vi "move_to_absolute_position.vi"(0 "device_index (in) [0=def]":i32, 5 "Error In":errorcluster) -> (19 "Error Out":errorcluster)   [LabVIEW 2013, in "examples.lvlib"]
doc: "Produced By:\n\n<B>Kod Integrations, LLC</B>\n4835 Marianne Drive\nMount Airy, MD 21771\nhttp://www.kodintegrations.com\nemail: info@kodintegrations.com\nphone: (240) 687-1288"
uses:
  libraries/examples.lvlib
  classes/Controller/_Controller.lvclass
  common/controls/motor_enabled_state_axes_group.ctl
  libraries/common.lvlib
  common/controls/axis.ctl
  common/controls/movement_item.ctl
panel:
  out "response":string
  out "success?":bool
  in  "target_value (in)":i32
  in  "axis (def=X)":T1
  in  "clear_buffer? (T)":bool=TRUE
  # "instructions:\n\nAt the specified device index, enter a target position\nvalue and (for multi-controller applications only) a\nspecific axis and run the VI.\n\nNOTE: This example VI makes an attempt to enable\nthe motor at the targeted axis.  If left disabled, the\nmove command will appear to be successful, but\nthe motor physically does not respond."
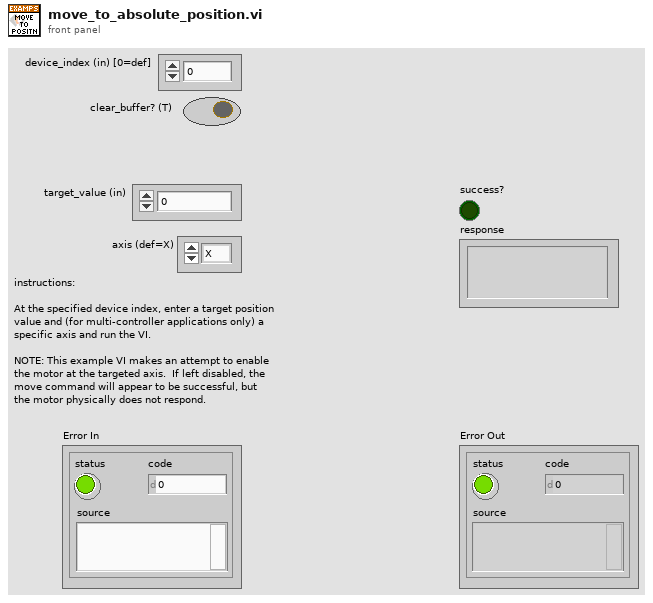
[diagram p1: front panel]
types:
  T1 = typedef "common.lvlib/axis.ctl" = enum16{"X", "Y", "Z", "U"}
  T2 = typedef "common.lvlib/movement_item.ctl" = cluster{"axis":T1, "target":i32}
  T3 = typedef "common.lvlib/motor_enabled_state_axes_group.ctl" = cluster{"x-axis":bool, "y-axis":bool, "z-axis":bool, "u-axis":bool}
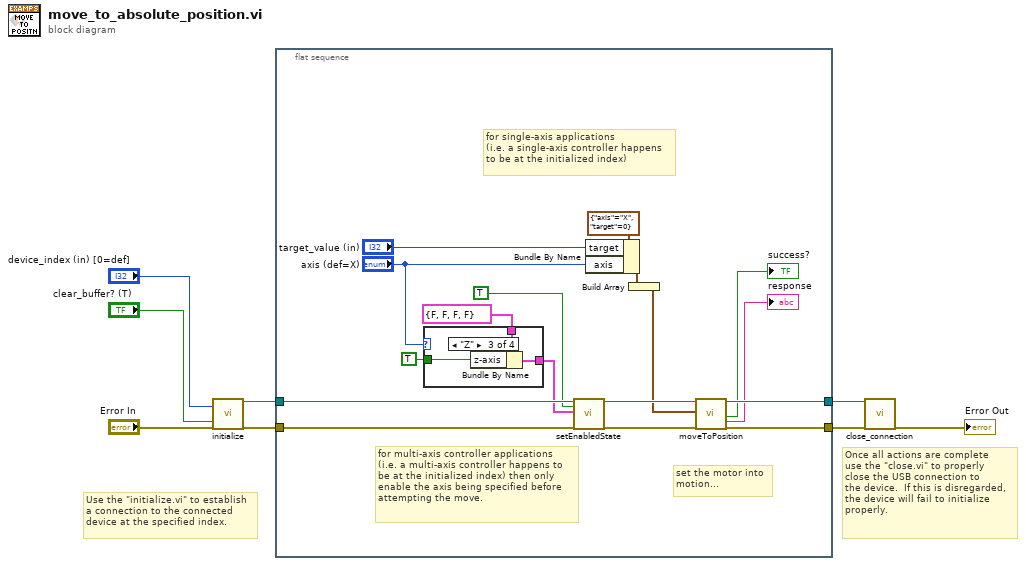
[diagram p0: block diagram]
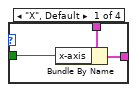
[diagram p2: hidden frame]
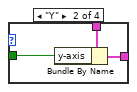
[diagram p3: hidden frame]
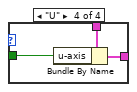
[diagram p4: hidden frame]
diagram:
  # "Once all actions are complete\nuse the \"close.vi\" to properly\nclose the USB connection to \nthe device.  If this is disregarded,\nthe device will fail to initialize \nproperly."
  # "Use the \"initialize.vi\" to establish\na connection to the connected\ndevice at the specified index."
  n1 = call "initialize.vi"("device_index (in) [0=def]"="device_index (in) [0=def]", "clear_buffer? (T)"="clear_buffer? (T)", "error in (no error)"="Error In") -> ("reference (out)"=w5:refnum<class "_Controller.lvclass">, "error out"=w4:errorcluster)  [unwired: 15 in]
  n2 = flat-sequence {
    tunnel: w5 -> [w21]
    tunnel: w4 -> [w20]
    tunnel: [w25] -> w3
    tunnel: [w24] -> w2
    frame #0 {
      # "set the motor into\nmotion..."
      # "for single-axis applications\n(i.e. a single-axis controller happens\nto be at the initialized index)"
      # "for multi-axis controller applications\n(i.e. a multi-axis controller happens to\nbe at the initialized index) then only \nenable the axis being specified before\nattempting the move."
      n3 = case shown="\"Z\"" "axis (def=X)" {
        tunnel: T3 {"x-axis"=FALSE, "y-axis"=FALSE, "z-axis"=FALSE, "u-axis"=FALSE} ("axes_states (for multi-axis applications only)") -> [w28 w31 w34 w37]
        tunnel: [w27 w30 w33 w36] -> w15
        tunnel: TRUE -> [w26 w29 w32 w35]
        frame "X", Default {
          n4 = Bundle By Name(cluster=w28, "x-axis"=w26) -> (w27:T3)
        }
        frame "Y" {
          n5 = Bundle By Name(cluster=w31, "y-axis"=w29) -> (w30:T3)
        }
        frame "Z" {
          n6 = Bundle By Name(cluster=w34, "z-axis"=w32) -> (w33:T3)
        }
        frame "U" {
          n7 = Bundle By Name(cluster=w37, "u-axis"=w35) -> (w36:T3)
        }
      }
      n8 = call-dynamic "setEnabledState.vi"("Controller in"=w21, "state (for single-axis applications only) - (def = DISABLED)"=TRUE ("state (for single-axis applications only)"), "axes_states (for multi-axis applications only) - (def = DISABLED)"=w15, "error in (no error)"=w20) -> ("Controller out"=w19:refnum<class "_Controller.lvclass">, "error out"=w18:errorcluster)  [unwired: 12 in, 2 out]
      n9 = Bundle By Name(cluster=T2 {"axis"=enum."X", "target"=0} ("item"), "target"="target_value (in)", "axis"="axis (def=X)") -> (w11:T2)
      n10 = Build Array(w11) -> (w9:T2[])
      n11 = call-dynamic "moveToPosition.vi"("Controller in"=w19, "target(s) (in)"=w9, "error in (no error)"=w18) -> ("Controller out"=w25:refnum<class "_Controller.lvclass">, "success?"=→"success?":bool, "response"=→"response":string, "error out"=w24:errorcluster)  [unwired: 13 in]
    }
  }
  n12 = call "close_connection.vi"("reference (in)"=w3, "error in (no error)"=w2) -> ("error out"=→"Error Out":errorcluster)  [unwired: 16 in, 1 out]
